vi "moveArc.vi"(0 "PMX4CXSAController in":refnum<class "PMX4CXSAController.lvclass">, 1 "x_coord":i32, 2 "y_coord":i32, 3 "direction":T1, 5 "error in (no error)":errorcluster, 7 "absolute_angle (degrees)":dbl, 9 "relative_angle (degrees)":dbl) -> (14 "PMX4CXSAController out":refnum<class "PMX4CXSAController.lvclass">, 17 "success?":bool, 18 "response":string, 19 "error out":errorcluster)   [LabVIEW 2020, in "classes.lvlib" / "PMX4CXSAController.lvclass"]
doc: "Produced By:\n\n<B>Kod Integrations, LLC</B>\n4835 Marianne Drive\nMount Airy, MD 21771\nhttp://www.kodintegrations.com\nemail: info@kodintegrations.com\nphone: (240) 687-1288"
uses:
  PMX4CXSAController.lvclass
  C:/GEECS/Developers Version/source/Device Drivers/Newmark-NSC-A/Arcus Driver 3.0.0/ArcusUsbComm/classes/Controller/_Controller.lvclass
  circular_direction.ctl
  _Controller.lvclass/_Controller.ctl
  _Controller.lvclass
  common.lvlib
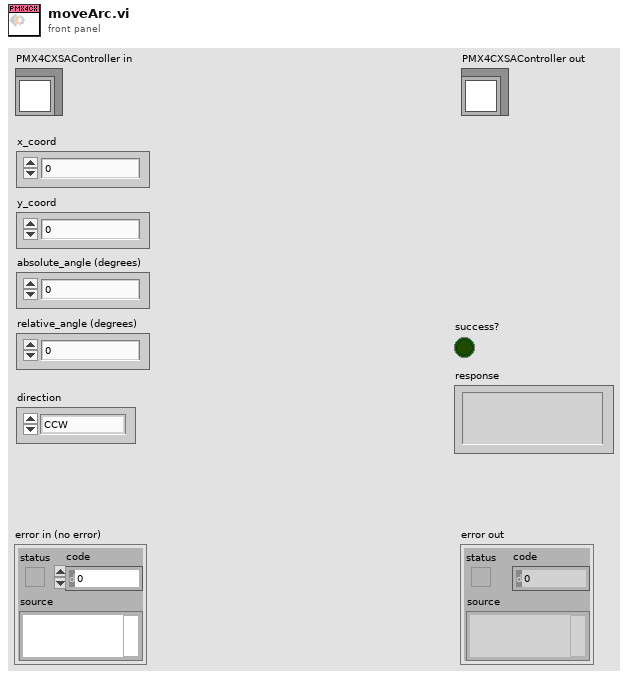
[diagram p1: front panel]
types:
  T1 = typedef "common.lvlib/circular_direction.ctl" = enum16{"CCW", "CW"}
  T2 = typedef "common.lvlib/models.ctl" = enum16{"<unrecognized>", "ACE-SDC", "ACE-SDE", "ACE-SXC", "ACE-SXE", "DMX-CAN", "DMX-J-SA", "DMX-K-SA", "DMX-UMD", "PMX-2ED-SA", "PMX-2EX-SA", "PMX-4CX-SA", "PMX-4EX-SA"}
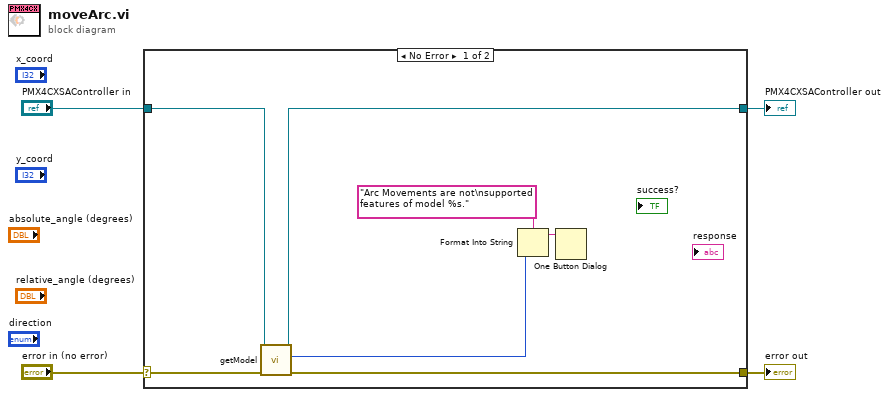
[diagram p0: block diagram]
diagram:
  n1 = case shown="No Error" "error in (no error)" {
    selector: "error in (no error)" -> [w8 w13]
    tunnel: [w7 w13] -> w3
    tunnel: [w5 w12] -> w1
    tunnel: "PMX4CXSAController in" -> [w6 w12]
    frame No Error {
      n2 = call "getModel.vi"("error in (no error)"=w8, "reference (in)"=w6) -> ("error out"=w7:errorcluster, "model"=w10:T2, "reference (out)"=w5:refnum<class "PMX4CXSAController.lvclass">)  [unwired: 7 in]
      n3 = Format Into String(format string="Arc Movements are not\nsupported features of model %s.", w10) -> (resulting string=w9:string)  [unwired: 2 in, 1 out]
      n4 = One Button Dialog(message=w9) -> ()  [unwired: 1 in, 1 out]
    }
    frame Error {
    }
  }
  "error out" <- w3
  "PMX4CXSAController out" <- w1
